vi "Get Redirection URL.vi"(8 "error in (no error)":errorcluster, 11 "HTTP GET Body":string) -> (0 "error out":errorcluster, 3 "Redirection URL":string)   [LabVIEW 2021, in "Web.lvlib"]
uses:
  Web.lvlib
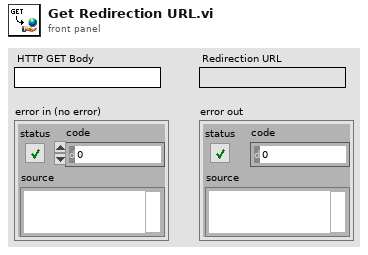
[diagram p1: front panel]
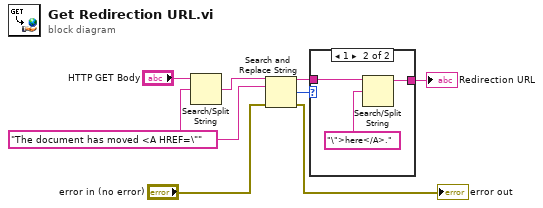
[diagram p0: block diagram]
diagram:
  w3 = "The document has moved <A HREF=\"" ("search string")
  n1 = Search/Split String(string="HTTP GET Body", search string/char (-)=w3) -> (match + rest of string=w8:string)  [unwired: 1 in, 2 out]
  n2 = Search and Replace String(input string=w8, search string=w3, error in="error in (no error)") -> (result string=w4:string, number of replacements=w1:i32, error out=→"error out":errorcluster)  [unwired: 5 in, 1 out]
  n3 = case shown="1" w1 {
    tunnel: [w9 w12] -> w7
    tunnel: w4 -> [w9 w10]
    frame 0, Default {
    }
    frame 1 {
      n4 = Search/Split String(string=w10, search string/char (-)="\">here</A>." ("search string")) -> (substring before match=w12:string)  [unwired: 1 in, 2 out]
    }
  }
  "Redirection URL" <- w7
